vi "Init UI.vi"(8 "error in (no error)":errorcluster, 11 "Editor in":refnum<class "Editor.lvclass">) -> (0 "error out":errorcluster, 3 "Editor out":refnum<class "Editor.lvclass">)   [LabVIEW 2020, in "VolatusGUIEditor.lvlib" / "Editor.lvclass"]
uses:
  Editor.lvclass
  Editor.lvclass/Editor.ctl
  Control List/Control List.lvclass
  lv-tree-tools/Tree Map/Tree Map/Tree Map.lvclass
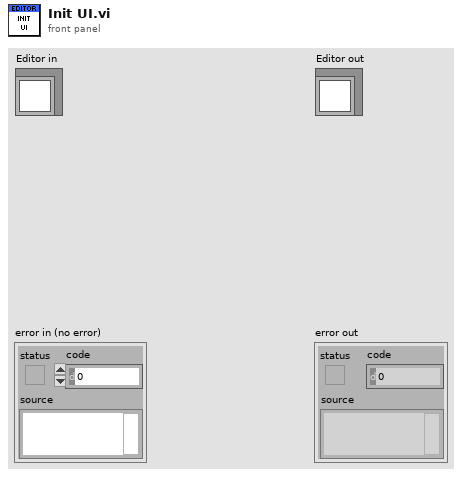
[diagram p1: front panel]
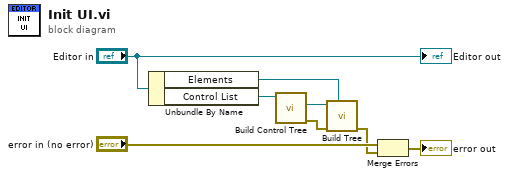
[diagram p0: block diagram]
diagram:
  n1 = Unbundle By Name("Editor in") -> ("Elements"=w5:refnum<vi>, "Control List"=w7:refnum<class "Control List.lvclass">)
  n2 = call "Build Control Tree.vi"("Control List in"=w7) -> ("error out"=w3:errorcluster, "Control Tree"=w6:refnum<class "Tree Map.lvclass">)  [unwired: 8 in, 1 out]
  n3 = call "Build Tree.vi"("Tree"=w5, "error in (no error)"=w3, "Tree Map in"=w6) -> ("error out"=w1:errorcluster)  [unwired: 7 in, 1 out]
  n4 = Merge Errors("error in (no error)", w1) -> (→"error out":errorcluster)
  "Editor out" <- "Editor in"
